vi "CompleteResourceUtilization.vi"() -> ()   [LabVIEW 2015]
uses:
  SingleAIConfig.ctl
  ScaleAndLimitAI16Config.ctl
  AI16LimitsConfig.ctl
  AI16ScaleConfig.ctl
  <vilib>/Platform/TimedLoop/XDataNode/timing_clust.ctl
  <vilib>/Platform/TimedLoop/XDataNode/nitl_modes.ctl
  <vilib>/Platform/TimedLoop/XDataNode/wakeup.ctl
  <vilib>/rvi/Emulation/niFpgaGetClockAttributes.vi
  <vilib>/rvi/Emulation/niFpgaSctlEmulationGetInTimedLoop.vi
  <vilib>/rvi/Emulation/niFpgaEmulationReportErrorSimple.vi
  <vilib>/rvi/eio/common/nirviEmuTemplateMethod_errors.vi
  <vilib>/rvi/Emulation/niFpgaCriticalErrorInLSC.vi
  <vilib>/eio/EIONode/EIONode.xnode
  <vilib>/Platform/TimedLoop/XDataNode/XDataNode.xnode
  <vilib>/Platform/TimedLoop/XDataNode/XDNodeRunTimeDep.lvlib
  ScaleAndLimit.lvlib
panel:
  in  "SingleAIConfig":T1
  out "loop time":u32
  out "AILimits":bool
  out "AILimitHigh":u16 format="%.0x"
  out "AILimitLow":u16 format="%.0x"
  in  "ClearLimits":bool
  out "ScaledAI":sgl[](array[numeric])
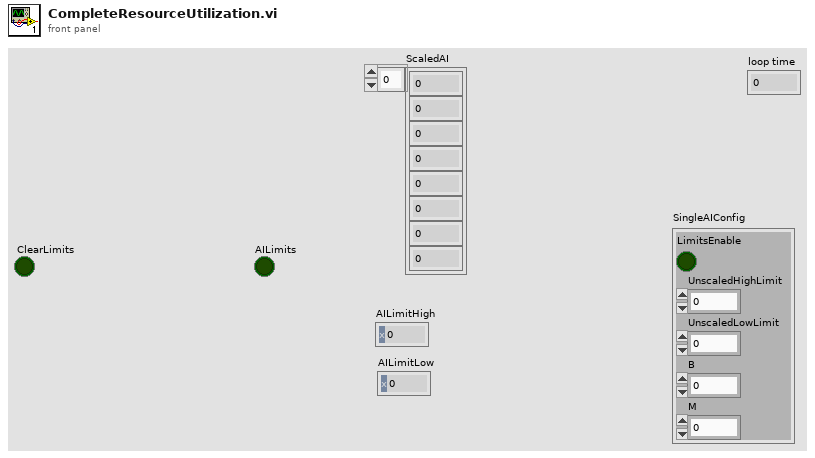
[diagram p1: front panel]
types:
  T1 = typedef "ScaleAndLimit.lvlib/SingleAIConfig.ctl" = cluster{"LimitsEnable":bool, "UnscaledHighLimit":i16, "UnscaledLowLimit":i16, "B":i16, "M":sgl}
  T2 = typedef "ScaleAndLimit.lvlib/ScaleAndLimitAI16Config.ctl" = cluster{"AI16Limits":T3, "AI16ScaleConfig":T4}
  T3 = typedef "ScaleAndLimit.lvlib/AI16LimitsConfig.ctl" = cluster{"LimitsEnabled":u16, "UnscaledHighLimit":i16[], "UnscaledLowLimit":i16[]}
  T4 = typedef "ScaleAndLimit.lvlib/AI16ScaleConfig.ctl" = cluster{"B":i16[], "M":sgl[]}
  T5 = typedef "XDNodeRunTimeDep.lvlib/timing_clust.ctl" = cluster{"Expected End [f-1]":u64, "Actual End [f-1]":u64, "Finished Late? [f-1]":bool, "Expected End [i-1]":u64, "Actual End [i-1]":u64, "Finished Late? [i-1]":bool, "Expected Start [i]":u64, "Actual Start [i]":u64, "Expected Start [f]":u64, "Actual Start [f]":u64, "Source Name":string, "Structure Name":string, "Period":i64, "Deadline":i64, "Offset":i64, "Start":i64, "Priority":i32, "Timeout":i32, "Mode":T6, "Wakeup Reason":T7, "Error":errorcluster, "Source Type":string, "Secondary Source Type":string, "Global End Time":u64, "Global Start Time":u64, "Frame Duration":u64, "Iteration Duration":u64, "Assigned CPU":i32, "I/O Scan Engine Mode":u32}
  T6 = typedef "XDNodeRunTimeDep.lvlib/nitl_modes.ctl" = enum32{"No Change", "Process missed periods, maintain original phase", "Discard missed periods, maintain original phase", "Process missed periods, ignore original phase", "Discard missed periods, ignore original phase"}
  T7 = typedef "XDNodeRunTimeDep.lvlib/wakeup.ctl" = enum32{"Normal", "Aborted", "Asynchronous wakeup", "Timing source error", "Timed loop error", "Timeout"}
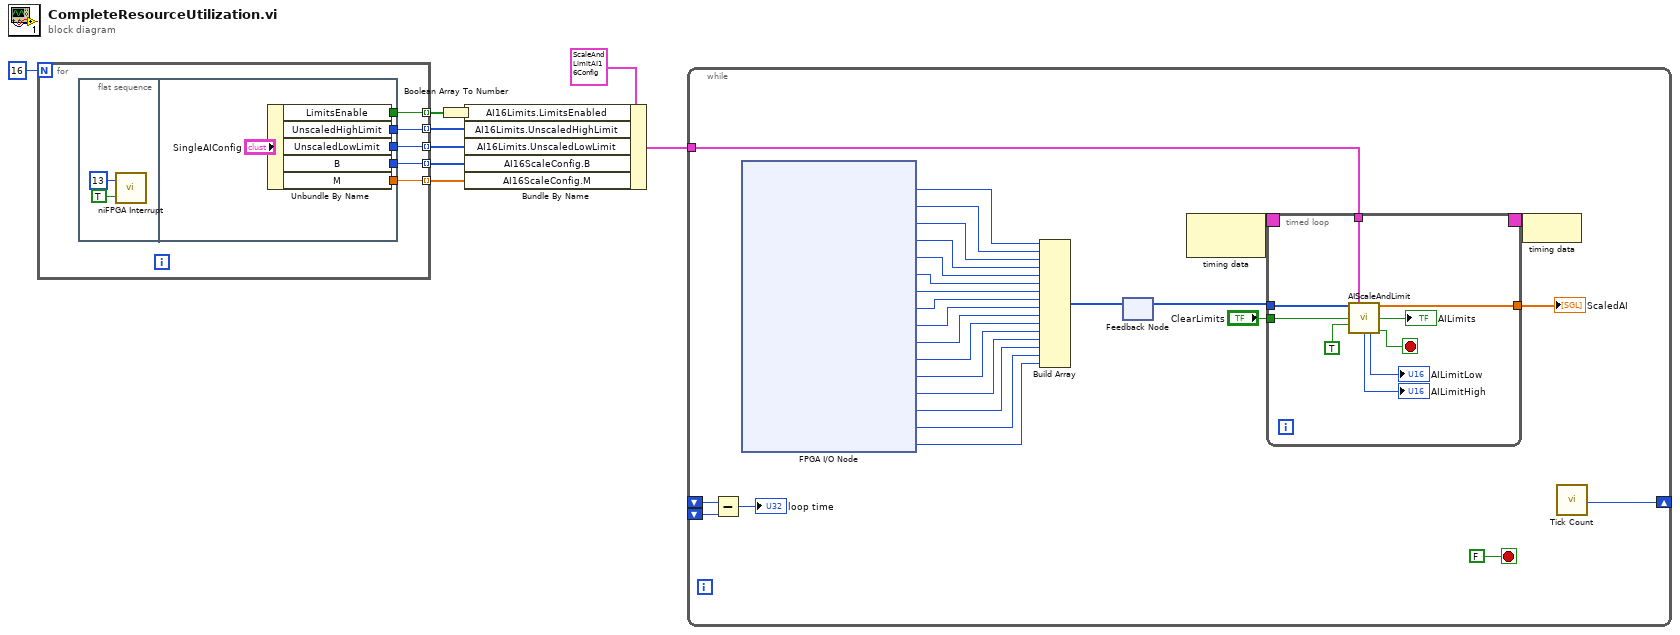
[diagram p0: block diagram]
diagram:
  n1 = for {
    N: 16 -> [_]
    tunnel: [w14] -> w7 mode=indexing
    tunnel: [w13] -> w4 mode=indexing
    tunnel: [w12] -> w3 mode=indexing
    tunnel: [w11] -> w2 mode=indexing
    tunnel: [w10] -> w1 mode=indexing
    n2 = flat-sequence {
      tunnel: [w21] -> w14
      tunnel: [w20] -> w13
      tunnel: [w19] -> w12
      tunnel: [w18] -> w11
      tunnel: [w17] -> w10
      frame #0 {
        n3 = call <vilib>:"niFPGA Interrupt.vi"("Wait Until Cleared (F)"=TRUE, "IRQ Number (0)"=u8 13) -> ()  [unwired: 1 in]
      }
      frame #1 {
        n4 = Unbundle By Name("SingleAIConfig") -> ("LimitsEnable"=w21:bool, "UnscaledHighLimit"=w20:i16, "UnscaledLowLimit"=w19:i16, "B"=w18:i16, "M"=w17:sgl)
      }
    }
  }
  n5 = Boolean Array To Number(Boolean array=w7) -> (number=w5:u16)
  n6 = Bundle By Name(cluster=T2 {"AI16Limits"={"LimitsEnabled"=0, "UnscaledHighLimit"=[0, 0, 0, 0, 0, 0, 0, 0, 0, 0, 0, 0, 0, 0, 0, 0], "UnscaledLowLimit"=[0, 0, 0, 0, 0, 0, 0, 0, 0, 0, 0, 0, 0, 0, 0, 0]}, "AI16ScaleConfig"={"B"=[0, 0, 0, 0, 0, 0, 0, 0, 0, 0, 0, 0, 0, 0, 0, 0], "M"=[0.0, 0.0, 0.0, 0.0, 0.0, 0.0, 0.0, 0.0, 0.0, 0.0, 0.0, 0.0, 0.0, 0.0, 0.0, 0.0]}} ("AIConfig"), "AI16Limits.LimitsEnabled"=w5, "AI16Limits.UnscaledHighLimit"=w4, "AI16Limits.UnscaledLowLimit"=w3, "AI16ScaleConfig.B"=w2, "AI16ScaleConfig.M"=w1) -> (w9:T2)
  n7 = while {
    shift-right: [w49] -> _
    shift-left: _ -> [w48]
    shift-left: _ -> [w47]
    tunnel: w9 -> [w45]
    stop <- FALSE stop-if-true
    n8 = Subtract(x=w48, y=w47) -> (x-y=→"loop time":u32)
    n9 = xnode "FPGA I/O Node"() -> ("RMC/Simultaneous/AI0"=w44:i16, "RMC/Simultaneous/AI1"=w43:i16, "RMC/Simultaneous/AI2"=w42:i16, "RMC/Simultaneous/AI3"=w41:i16, "RMC/Simultaneous/AI4"=w40:i16, "RMC/Simultaneous/AI5"=w39:i16, "RMC/Simultaneous/AI6"=w38:i16, "RMC/Simultaneous/AI7"=w37:i16, "RMC/Simultaneous/AI8"=w36:i16, "RMC/Simultaneous/AI9"=w35:i16, "RMC/Simultaneous/AI10"=w34:i16, "RMC/Simultaneous/AI11"=w33:i16, "RMC/Simultaneous/AI12"=w32:i16, "RMC/Simultaneous/AI13"=w31:i16, "RMC/Simultaneous/AI14"=w30:i16, "RMC/Simultaneous/AI15"=w29:i16)  [unwired: 16 in, 16 out]
    n10 = Build Array(w44, w43, w42, w41, w40, w39, w38, w37, w36, w35, w34, w33, w32, w31, w30, w29) -> (w24:i16[])
    n11 = feedback-in #1(w24) -> ()
    n12 = feedback #1() -> (w23:i16[])  [unwired: 1 in]
    n13 = node-c288() -> (w28:T5)  [unwired: 1 in]
    n14 = timed-loop {
      timing: w28 -> [_]
      timing-out: [_] -> w27
      tunnel: w23 -> [w59]
      tunnel: w45 -> [w51]
      tunnel: "ClearLimits" -> [w58]
      tunnel: [w56] -> w26
      stop <- w54 stop-if-true
      n15 = call "AIScaleAndLimit.vi"("UnscaledAI"=w59, "RawAIConfig"=w51, "ClearLimits"=w58, "input valid"=TRUE) -> ("ScaledAI"=w56:sgl[], "AILimits"=→"AILimits":bool, "AILimitHigh"=→"AILimitHigh":u16, "ALimitLow"=→"AILimitLow":u16, "output valid"=w54:bool)  [unwired: 6 in, 1 out]
    }
    "ScaledAI" <- w26
    n16 = node-c288(w27) -> ()
    n17 = call "Tick Count"() -> ("Tick Count(Ticks)"=w49:u32)
  }
